vi "GV-SetYstdScale.vi"(8 "error in (no error)":errorcluster, 11 "Gviewer in":refnum<class "Gviewer.lvclass">) -> (0 "error out":errorcluster, 3 "Gviewer out":refnum<class "Gviewer.lvclass">)   [LabVIEW 2020, in "Sgraph_lib_V1.lvlib" / "Gviewer.lvclass"]
doc: "Andre Koelewijn, 30 jan 2021\n\nAdapt the Standard Y scale to one of the TAGs"
uses:
  Gviewer.lvclass
  Gviewer.lvclass/Gviewer.ctl
  controls/Typedef_Gserver-Replies.ctl
  controls/Typedef_ServerActions.ctl
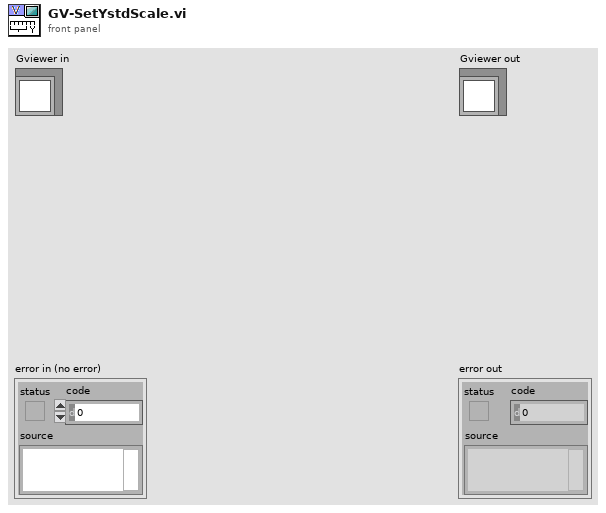
[diagram p1: front panel]
types:
  T1 = typedef "Sgraph_lib_V1.lvlib/Gviewer.lvclass/Typedef_ServerActions.ctl" = enum16{"GraphUpdate", "SendAllTags", "SendIniPath", "SetGeneralOptions", "EditTagsOpen", "EditTagsPresetSave", "EditTagsPresetLoad", "EditTagsClose", "NewTagSelection", "AutoScale", "DBeditStatus", "DBsaveConfirm", "ExitGraph"}
  T2 = typedef "Typedef_Gserver-Replies.ctl" = cluster{"ServerActions":T1, "data":variant, "Source":string, "Time Stamp":timestamp}
  T3 = typedef "Sgraph_lib_V1.lvlib/Gviewer.lvclass/Typedef_SelProperties.ctl" = cluster{"Color":u32, "LineType":T4, "max":dbl, "min":dbl, "unit":string}
  T4 = typedef "Sgraph_lib_V1.lvlib/Gviewer.lvclass/Typedef_LineType.ctl" = enum16{"num_bare", "num_MinMax_Area", "num_MinMax_Lines", "num_MinMax_Forfor", "num_Max_Area", "num_Max_Line", "num_Max_Forfor", "num_Min_Area", "num_Min_Line", "num_Min_Fosfor", "Boolean_Line_01", "Boolean_Area_01", "Boolean_Fosfor_01", "Boolean_Line_TF", "Boolean_Area_TF", "Boolean_Fosfor_TF", "Boolean_OnOff_Line", "Boolean_OnOff_Area", "Boolean_OnOff_Fosfor", "Boolean_spare", "StringEvent_Line", "StringEvent_TimeLine"}
  T5 = typedef "Sgraph_lib_V1.lvlib/FAMM.lvclass/FAMM_reply_datagram.ctl" = cluster{"GraphName":string, "Time-Start":timestamp, "Time-End":timestamp, "TimeSpan":dbl, "Live":T6, "WAQ_section":T7, "EAQ_section":T8, "PAQ_section":T9, "Layer":i32}
  T6 = typedef "Sgraph_lib_V1.lvlib/Gviewer.lvclass/Typedef_Live.ctl" = enum16{"Live View", "Freeze"}
  T7 = typedef "Sgraph_lib_V1.lvlib/FAMM.lvclass/FAMM_reply_WAQdata.ctl" = cluster{"Boolean":bool}
  T8 = typedef "Sgraph_lib_V1.lvlib/FAMM.lvclass/FAMM_reply_EAQdata.ctl" = cluster{"Boolean":bool}
  T9 = typedef "Sgraph_lib_V1.lvlib/FAMM.lvclass/FAMM_reply_PAQdata.ctl" = cluster{"Tags":string[], "time stamp":timestamp[], "DataSection":cluster{"data":dbl[], "max":dbl[], "min":dbl[], "Status":u32[]}[]}
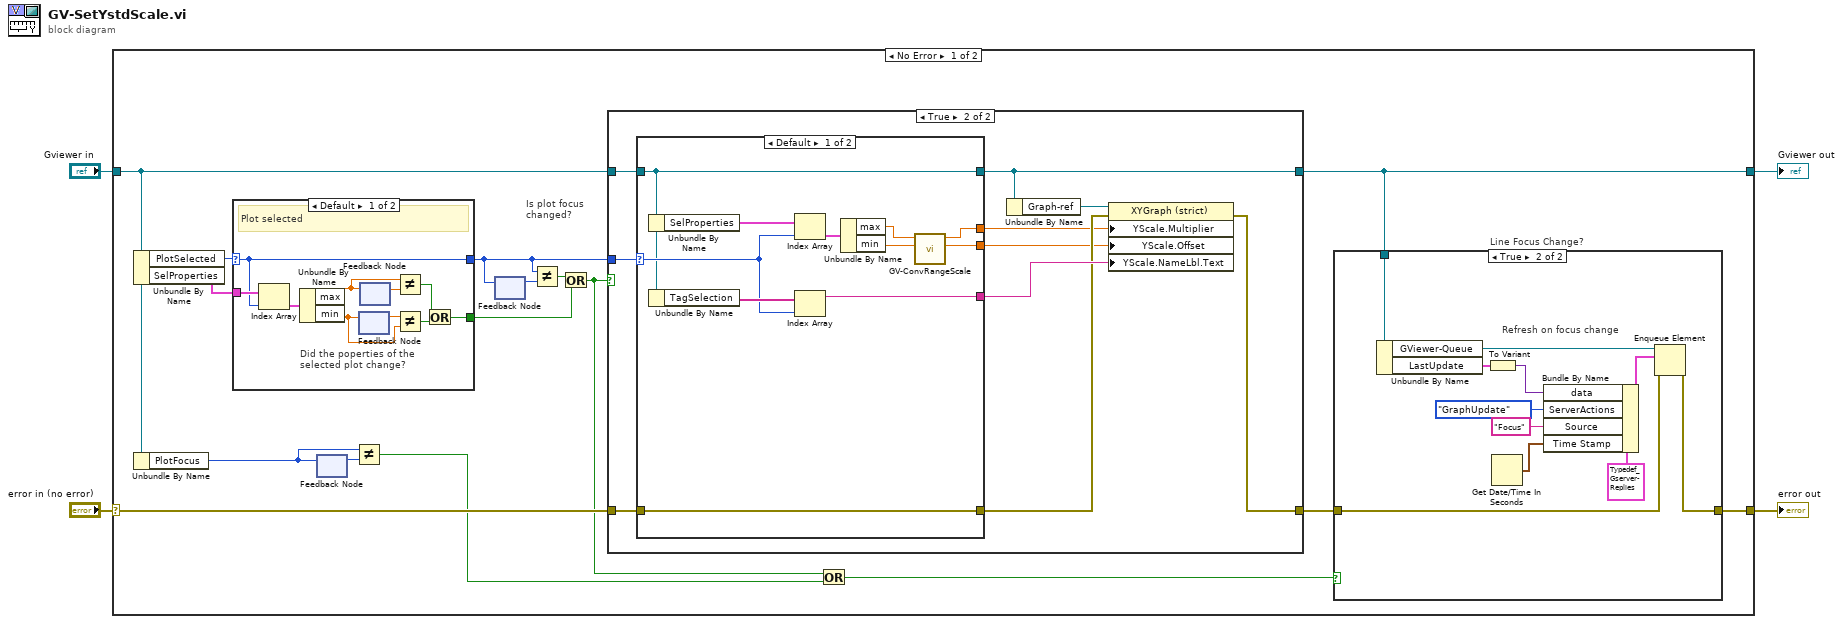
[diagram p0: block diagram]
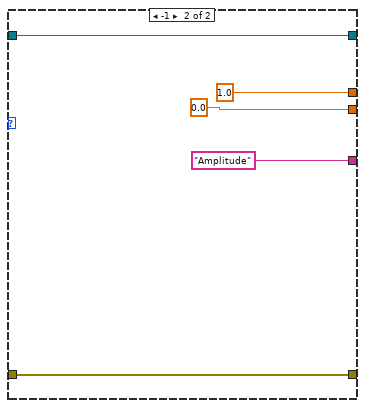
[diagram p4: hidden frame]
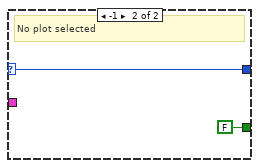
[diagram p5: hidden frame]
diagram:
  n1 = case shown="No Error" "error in (no error)" {
    selector: "error in (no error)" -> [w19 w74]
    tunnel: [w6 w74] -> w3
    tunnel: [w5 w73] -> w1
    tunnel: "Gviewer in" -> [w12 w73]
    frame No Error {
      # "Is plot focus\nchanged?"
      n2 = Unbundle By Name(w12) -> ("PlotSelected"=w20:i32, "SelProperties"=w15:T3[])
      n3 = Unbundle By Name(w12) -> ("PlotFocus"=w11:i32)
      n4 = case shown="Default" w20 {
        selector: w20 -> [w61 w71]
        tunnel: [w61 w71] -> w17
        tunnel: w15 -> [w70 _]
        tunnel: [w62 FALSE] -> w14
        frame Default {
          # "Did the poperties of the\nselected plot change?"
          # "Plot selected"
          n5 = Index Array(array=w70, index=w61) -> (element=w69:T3)
          n6 = Unbundle By Name(w69) -> ("max"=w67:dbl, "min"=w65:dbl)
          n7 = feedback #1() -> (w66:dbl)  [unwired: 1 in]
          n8 = feedback-in #1(w65) -> ()
          n9 = feedback #2() -> (w68:dbl)  [unwired: 1 in]
          n10 = feedback-in #2(w67) -> ()
          n11 = Not Equal?(x=w67, y=w68) -> (x != y?=w64:bool)
          n12 = Not Equal?(x=w66, y=w65) -> (x != y?=w63:bool)
          n13 = Or(x=w64, y=w63) -> (x .or. y?=w62:bool)
        }
        frame -1 {
          # "No plot selected"
        }
      }
      n14 = feedback #3() -> (w13:i32)  [unwired: 1 in]
      n15 = feedback-in #3(w11) -> ()
      n16 = Not Equal?(x=w11, y=w13) -> (x != y?=w9:bool)
      n17 = feedback-in #4(w17) -> ()
      n18 = feedback #4() -> (w18:i32)  [unwired: 1 in]
      n19 = Not Equal?(x=w17, y=w18) -> (x != y?=w16:bool)
      n20 = Or(x=w16, y=w14) -> (x .or. y?=w10:bool)
      n21 = case shown="True" w10 {
        tunnel: w17 -> [_ w44]
        tunnel: w12 -> [w33 w43]
        tunnel: w19 -> [w34 w42]
        tunnel: [w33 w35] -> w5
        tunnel: [w34 w38] -> w7
        frame False {
        }
        frame True {
          n22 = case shown="Default" w44 {
            selector: w44 -> [w50 _]
            tunnel: w43 -> [w46 w60]
            tunnel: w42 -> [w45 w59]
            tunnel: [w46 w60] -> w35
            tunnel: [w45 w59] -> w39
            tunnel: [w48 1.0] -> w37
            tunnel: [w47 0.0] -> w36
            tunnel: [w49 "Amplitude" ("Tag")] -> w40
            frame Default {
              n23 = Unbundle By Name(w46) -> ("SelProperties"=w55:T3[])
              n24 = Unbundle By Name(w46) -> ("TagSelection"=w51:string[])
              n25 = Index Array(array=w55, index=w50) -> (element=w54:T3)
              n26 = Index Array(array=w51, index=w50) -> (element=w49:string)
              n27 = Unbundle By Name(w54) -> ("max"=w52:dbl, "min"=w53:dbl)
              n28 = call "GV-ConvRangeScale.vi"("RangeL"=w53, "RangeH"=w52) -> ("Offset"=w47:dbl, "Gain"=w48:dbl)  [unwired: 8 in]
            }
            frame -1 {
            }
          }
          n29 = Unbundle By Name(w35) -> ("Graph-ref"=w41:refnum<vi>)
          n30 = property class="XYGraph (strict)"(reference=w41, error in=w39, "YScale.Multiplier"=w37, "YScale.Offset"=w36, "YScale.NameLbl.Text"=w40) -> (error out=w38:errorcluster)  [unwired: 1 out]
        }
      }
      n31 = Or(x=w10, y=w9) -> (x .or. y?=w8:bool)
      n32 = case "Line Focus Change?" shown="True" w8 {
        tunnel: w7 -> [w21 w24]
        tunnel: [w21 w23] -> w6
        tunnel: w5 -> [_ w22]
        frame False {
        }
        frame True {
          # "Refresh on focus change"
          n33 = Unbundle By Name(w22) -> ("GViewer-Queue"=w32:refnum<queue>, "LastUpdate"=w30:T5)
          n34 = To Variant(anything=w30) -> (Variant=w29:variant)
          n35 = Get Date/Time In Seconds() -> (seconds since 1Jan1904=w31:timestamp)
          n36 = Bundle By Name(cluster=T2 {"ServerActions"=enum."GraphUpdate", "data"=variant, "Source"="", "Time Stamp"=timestamp(0 s since 1904-01-01)} ("element"), "data"=w29, "ServerActions"=Typedef_ServerActions."GraphUpdate", "Source"="Focus", "Time Stamp"=w31) -> (w28:T2)
          n37 = Enqueue Element(queue=w32, element=w28, error in (no error)=w24) -> (error out=w23:errorcluster)  [unwired: 1 in, 2 out]
        }
      }
    }
    frame Error {
    }
  }
  "error out" <- w3
  "Gviewer out" <- w1
